vi "战舰+敌机爆炸.vi"() -> ()   [LabVIEW 2018]
panel:
  out "敌机爆炸":picture
  in  "敌机数量":dbl
  in  "敌机速度":dbl
  out "敌机":picture
  out "按键":dbl
  out "战舰":T1
  out "激光武器1":T2
  out "激光武器 2":T2
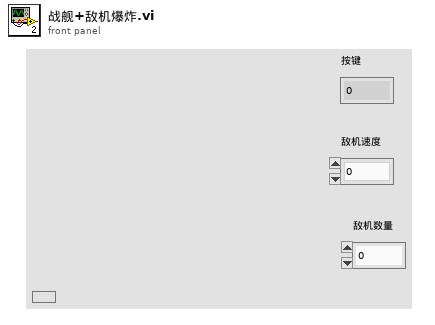
[diagram p1: front panel]
types:
  T1 = typedef "战列巡洋舰.ctl" = picture
  T2 = typedef "战列巡洋舰_激光武器.ctl" = picture
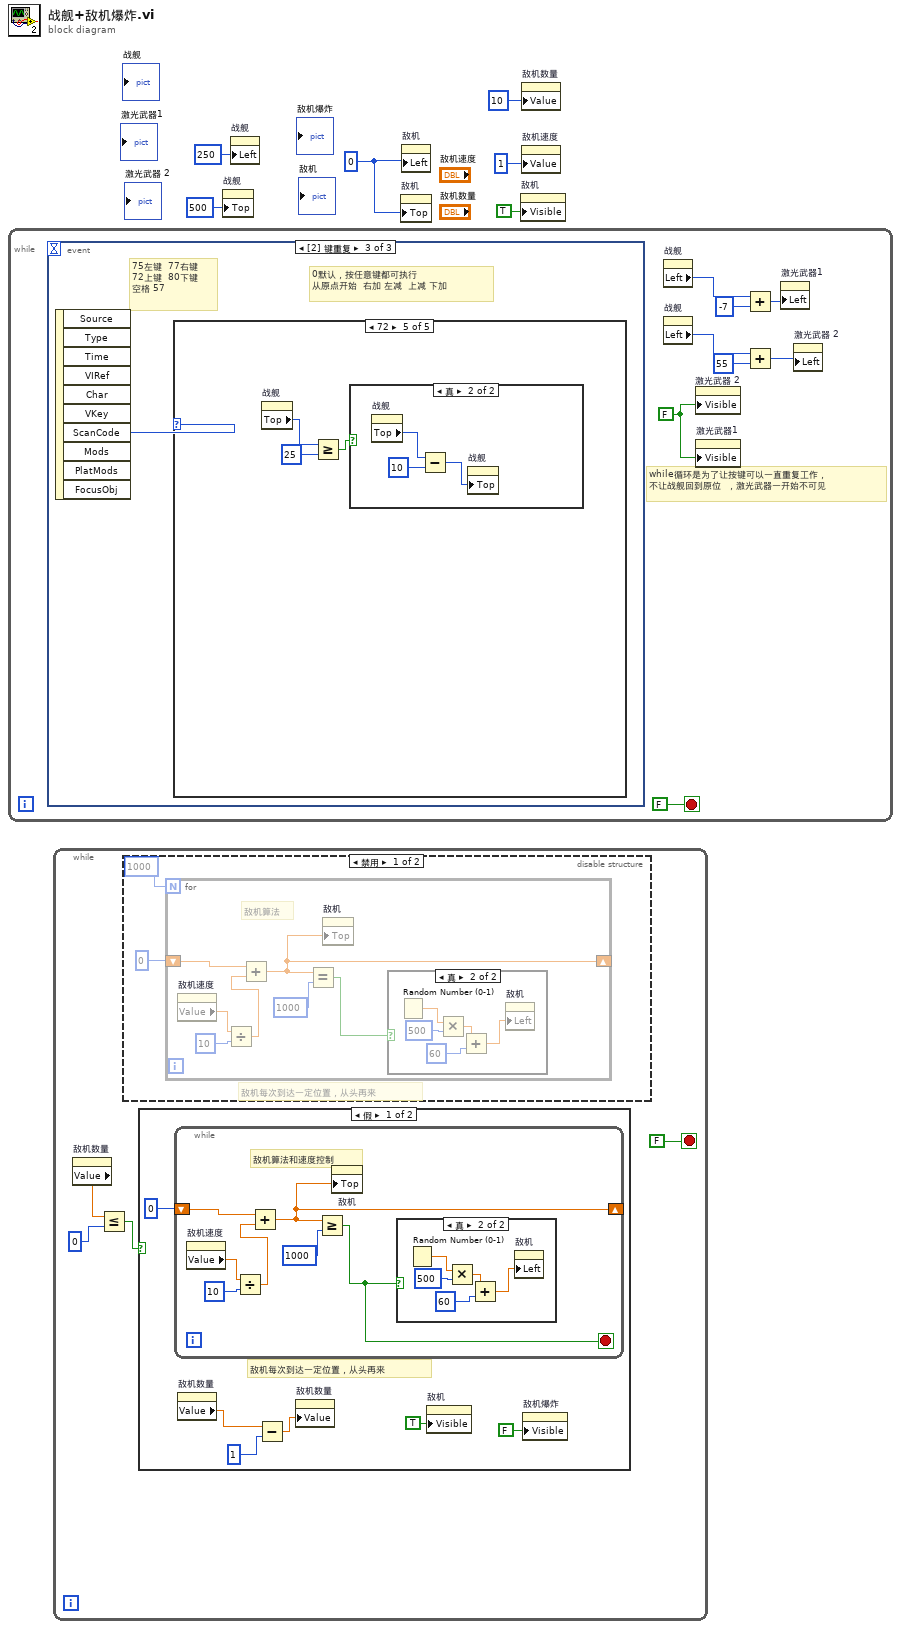
[diagram p0: block diagram]
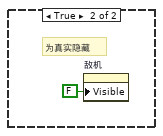
[diagram p3: hidden frame]
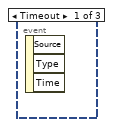
[diagram p6: hidden frame]
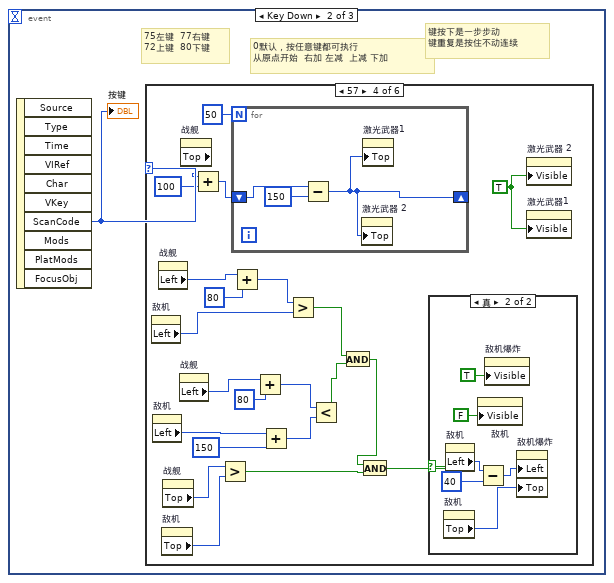
[diagram p7: hidden frame]
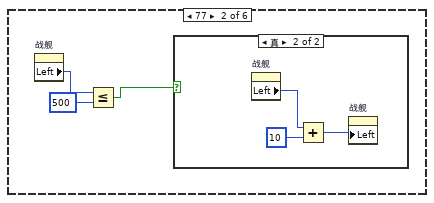
[diagram p9: hidden frame]
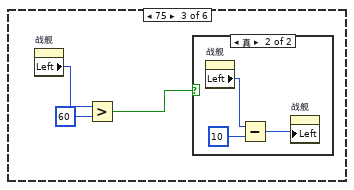
[diagram p11: hidden frame]
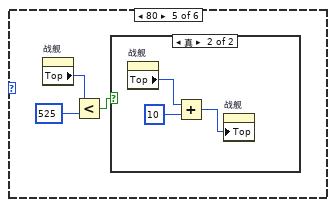
[diagram p14: hidden frame]
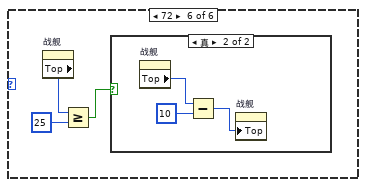
[diagram p16: hidden frame]
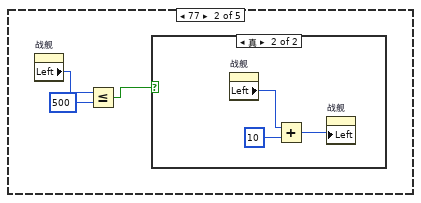
[diagram p19: hidden frame]
diagram:
  w1 = 0
  n1 = while {
    stop <- FALSE stop-if-true
    w7 = FALSE
    # "while循环是为了让按键可以一直重复工作，\n不让战舰回到原位  ，激光武器一开始不可见"
    n2 = event shown="[2] 键重复" {
      selector: _ -> [_ _ _]
      dyn-events: _ -> [_ _ _]
      timeout: _ -> [_ _ _]
      event Timeout {
        n3 = event-data() -> ()  [unwired: 1 in, 3 out]
      }
      event Key Down {
        # "键按下是一步步动\n键重复是按住不动连续"
        # "75左键  77右键\n72上键  80下键"
        # "0默认，按任意键都可执行\n从原点开始  右加 左减  上减 下加"
        n4 = event-data() -> ("ScanCode"=w15:i16)  [unwired: 1 in, 9 out]
        "按键" <- w15
        n5 = case shown="57" w15 {
          frame 0, Default {
          }
          frame 77 {
            n6 = property on="战舰" class="Pict (严格)"() -> ("Left"=w18:i32)  [unwired: 2 in, 2 out]
            n7 = Less Or Equal?(x=w18, y=500) -> (x <= y?=w16:bool)
            n8 = case shown="真" w16 {
              frame False {
              }
              frame True {
                n9 = property on="战舰" class="Pict (严格)"() -> ("Left"=w20:i32)  [unwired: 2 in, 2 out]
                n10 = Add(x=w20, y=10) -> (x+y=w21:i32)
                n11 = property on="战舰" class="Pict (严格)"("Left"=w21) -> ()  [unwired: 2 in, 2 out]
              }
            }
          }
          frame 75 {
            n12 = property on="战舰" class="Pict (严格)"() -> ("Left"=w24:i32)  [unwired: 2 in, 2 out]
            n13 = Greater?(x=w24, y=60) -> (0:w22:bool)
            n14 = case shown="真" w22 {
              frame False {
              }
              frame True {
                n15 = property on="战舰" class="Pict (严格)"() -> ("Left"=w26:i32)  [unwired: 2 in, 2 out]
                n16 = Subtract(x=w26, y=10) -> (x-y=w27:i32)
                n17 = property on="战舰" class="Pict (严格)"("Left"=w27) -> ()  [unwired: 2 in, 2 out]
              }
            }
          }
          frame 57 {
            w45 = TRUE
            n18 = property on="敌机" class="Pict"() -> ("Left"=w42:i32)  [unwired: 2 in, 2 out]
            n19 = property on="敌机" class="Pict"() -> ("Left"=w35:i32)  [unwired: 2 in, 2 out]
            n20 = property on="战舰" class="Pict (严格)"() -> ("Left"=w44:i32)  [unwired: 2 in, 2 out]
            n21 = property on="敌机" class="Pict"() -> ("Top"=w28:i32)  [unwired: 2 in, 2 out]
            n22 = property on="战舰" class="Pict (严格)"() -> ("Top"=w29:i32)  [unwired: 2 in, 2 out]
            n23 = property on="战舰" class="Pict (严格)"() -> ("Left"=w37:i32)  [unwired: 2 in, 2 out]
            n24 = property on="战舰" class="Pict (严格)"() -> ("Top"=w48:i32)  [unwired: 2 in, 2 out]
            n25 = Add(x=w48, y=100) -> (x+y=w46:i32)
            n26 = Greater?(x=w29, y=w28) -> (0:w31:bool)
            n27 = for {
              N: 50 -> [_]
              shift-right: [w56] -> _
              shift-left: w46 -> [w58]
              n28 = Subtract(x=w58, y=150) -> (x-y=w56:i32)
              n29 = property on="激光武器 2" class="Pict (严格)"("Top"=w56) -> ()  [unwired: 2 in, 2 out]
              n30 = property on="激光武器1" class="Pict (严格)"("Top"=w56) -> ()  [unwired: 2 in, 2 out]
            }
            n31 = Add(x=w44, y=80) -> (x+y=w41:i32)
            n32 = Add(x=w37, y=80) -> (x+y=w39:i32)
            n33 = Add(x=w35, y=150) -> (x+y=w34:i32)
            n34 = Greater?(x=w41, y=w42) -> (0:w40:bool)
            n35 = Less?(x=w39, y=w34) -> (x < y?=w36:bool)
            n36 = And(x=w40, y=w36) -> (x .and. y?=w32:bool)
            n37 = And(x=w32, y=w31) -> (x .and. y?=w30:bool)
            n38 = case shown="真" w30 {
              frame False {
              }
              frame True {
                n39 = property on="敌机" class="Pict"() -> ("Top"=w53:i32)  [unwired: 2 in, 2 out]
                n40 = property on="敌机" class="Pict"() -> ("Left"=w51:i32)  [unwired: 2 in, 2 out]
                n41 = property on="敌机" class="Pict"("Visible"=FALSE ("可见")) -> ()  [unwired: 2 in, 2 out]
                n42 = Subtract(x=w51, y=40) -> (x-y=w50:i32)
                n43 = property on="敌机爆炸" class="Pict"("Visible"=TRUE ("可见")) -> ()  [unwired: 2 in, 2 out]
                n44 = property on="敌机爆炸" class="Pict"("Left"=w50, "Top"=w53) -> ()  [unwired: 2 in, 2 out]
              }
            }
            n45 = property on="激光武器 2" class="Pict (严格)"("Visible"=w45) -> ()  [unwired: 2 in, 2 out]
            n46 = property on="激光武器1" class="Pict (严格)"("Visible"=w45) -> ()  [unwired: 2 in, 2 out]
          }
          frame 80 {
            n47 = property on="战舰" class="Pict (严格)"() -> ("Top"=w61:i32)  [unwired: 2 in, 2 out]
            n48 = Less?(x=w61, y=525) -> (x < y?=w59:bool)
            n49 = case shown="真" w59 {
              frame False {
              }
              frame True {
                n50 = property on="战舰" class="Pict (严格)"() -> ("Top"=w63:i32)  [unwired: 2 in, 2 out]
                n51 = Add(x=w63, y=10) -> (x+y=w62:i32)
                n52 = property on="战舰" class="Pict (严格)"("Top"=w62) -> ()  [unwired: 2 in, 2 out]
              }
            }
          }
          frame 72 {
            n53 = property on="战舰" class="Pict (严格)"() -> ("Top"=w67:i32)  [unwired: 2 in, 2 out]
            n54 = Greater Or Equal?(x=w67, y=25) -> (x >= y?=w66:bool)
            n55 = case shown="真" w66 {
              frame False {
              }
              frame True {
                n56 = property on="战舰" class="Pict (严格)"() -> ("Top"=w70:i32)  [unwired: 2 in, 2 out]
                n57 = Subtract(x=w70, y=10) -> (x-y=w69:i32)
                n58 = property on="战舰" class="Pict (严格)"("Top"=w69) -> ()  [unwired: 2 in, 2 out]
              }
            }
          }
        }
      }
      event Key Repeat {
        # "75左键  77右键\n72上键  80下键\n空格 57"
        # "0默认，按任意键都可执行\n从原点开始  右加 左减  上减 下加"
        n59 = event-data() -> ("ScanCode"=w71:i16)  [unwired: 1 in, 9 out]
        n60 = case shown="72" w71 {
          frame 0, Default {
          }
          frame 77 {
            n61 = property on="战舰" class="Pict (严格)"() -> ("Left"=w74:i32)  [unwired: 2 in, 2 out]
            n62 = Less Or Equal?(x=w74, y=500) -> (x <= y?=w73:bool)
            n63 = case shown="真" w73 {
              frame False {
              }
              frame True {
                n64 = property on="战舰" class="Pict (严格)"() -> ("Left"=w76:i32)  [unwired: 2 in, 2 out]
                n65 = Add(x=w76, y=10) -> (x+y=w77:i32)
                n66 = property on="战舰" class="Pict (严格)"("Left"=w77) -> ()  [unwired: 2 in, 2 out]
              }
            }
          }
          frame 75 {
            n67 = property on="战舰" class="Pict (严格)"() -> ("Left"=w80:i32)  [unwired: 2 in, 2 out]
            n68 = Greater Or Equal?(x=w80, y=25) -> (x >= y?=w79:bool)
            n69 = case shown="真" w79 {
              frame False {
              }
              frame True {
                n70 = property on="战舰" class="Pict (严格)"() -> ("Left"=w83:i32)  [unwired: 2 in, 2 out]
                n71 = Subtract(x=w83, y=10) -> (x-y=w82:i32)
                n72 = property on="战舰" class="Pict (严格)"("Left"=w82) -> ()  [unwired: 2 in, 2 out]
              }
            }
          }
          frame 80 {
            n73 = property on="战舰" class="Pict (严格)"() -> ("Top"=w86:i32)  [unwired: 2 in, 2 out]
            n74 = Less Or Equal?(x=w86, y=525) -> (x <= y?=w85:bool)
            n75 = case shown="真" w85 {
              frame False {
              }
              frame True {
                n76 = property on="战舰" class="Pict (严格)"() -> ("Top"=w88:i32)  [unwired: 2 in, 2 out]
                n77 = Add(x=w88, y=10) -> (x+y=w87:i32)
                n78 = property on="战舰" class="Pict (严格)"("Top"=w87) -> ()  [unwired: 2 in, 2 out]
              }
            }
          }
          frame 72 {
            n79 = property on="战舰" class="Pict (严格)"() -> ("Top"=w92:i32)  [unwired: 2 in, 2 out]
            n80 = Greater Or Equal?(x=w92, y=25) -> (x >= y?=w91:bool)
            n81 = case shown="真" w91 {
              frame False {
              }
              frame True {
                n82 = property on="战舰" class="Pict (严格)"() -> ("Top"=w95:i32)  [unwired: 2 in, 2 out]
                n83 = Subtract(x=w95, y=10) -> (x-y=w94:i32)
                n84 = property on="战舰" class="Pict (严格)"("Top"=w94) -> ()  [unwired: 2 in, 2 out]
              }
            }
          }
        }
      }
    }
    n85 = property on="战舰" class="Pict (严格)"() -> ("Left"=w13:i32)  [unwired: 2 in, 2 out]
    n86 = property on="战舰" class="Pict (严格)"() -> ("Left"=w9:i32)  [unwired: 2 in, 2 out]
    n87 = property on="激光武器 2" class="Pict (严格)"("Visible"=w7) -> ()  [unwired: 2 in, 2 out]
    n88 = property on="激光武器1" class="Pict (严格)"("Visible"=w7) -> ()  [unwired: 2 in, 2 out]
    n89 = Add(x=w13, y=-7) -> (x+y=w12:i32)
    n90 = Add(x=w9, y=55) -> (x+y=w8:i32)
    n91 = property on="激光武器1" class="Pict (严格)"("Left"=w12) -> ()  [unwired: 2 in, 2 out]
    n92 = property on="激光武器 2" class="Pict (严格)"("Left"=w8) -> ()  [unwired: 2 in, 2 out]
  }
  n93 = while {
    stop <- FALSE stop-if-true
    n94 = property on="敌机数量" class="DigNum (严格)"() -> ("Value"=w98:dbl)  [unwired: 2 in, 2 out]
    n95 = Less Or Equal?(x=w98, y=0) -> (x <= y?=w97:bool)
    n96 = disable-structure shown="禁用" {
      frame Disabled {
        # "敌机每次到达一定位置，从头再来"
        n97 = for {
          N: 1000 -> [_]
          shift-right: [w124] -> _
          shift-left: 0 -> [w127]
          # "敌机算法"
          n98 = property on="敌机速度" class="DigNum (严格)"() -> ("Value"=w123:dbl)  [unwired: 2 in, 2 out]
          n99 = Divide(x=w123, y=10) -> (x/y=w122:dbl)
          n100 = Add(x=w127, y=w122) -> (x+y=w124:dbl)
          n101 = Equal?(x=w124, y=1000) -> (x = y?=w125:bool)
          n102 = property on="敌机" class="Pict"("Top"=w124) -> ()  [unwired: 2 in, 2 out]
          n103 = case shown="真" w125 {
            frame False {
            }
            frame True {
              n104 = Random Number (0-1)() -> (number: 0 to 1=w132:dbl)
              n105 = Multiply(x=w132, y=500) -> (x*y=w130:dbl)
              n106 = Add(x=w130, y=60) -> (x+y=w129:dbl)
              n107 = property on="敌机" class="Pict"("Left"=w129) -> ()  [unwired: 2 in, 2 out]
            }
          }
        }
      }
      frame Enabled {
      }
    }
    n108 = case shown="假" w97 {
      frame False {
        # "敌机每次到达一定位置，从头再来"
        n109 = while {
          shift-right: [w110] -> _
          shift-left: 0 -> [w112]
          stop <- w106 stop-if-true
          # "敌机算法和速度控制"
          n110 = property on="敌机速度" class="DigNum (严格)"() -> ("Value"=w109:dbl)  [unwired: 2 in, 2 out]
          n111 = Divide(x=w109, y=10) -> (x/y=w108:dbl)
          n112 = Add(x=w112, y=w108) -> (x+y=w110:dbl)
          n113 = Greater Or Equal?(x=w110, y=1000) -> (x >= y?=w106:bool)
          n114 = property on="敌机" class="Pict"("Top"=w110) -> ()  [unwired: 2 in, 2 out]
          n115 = case shown="真" w106 {
            frame False {
            }
            frame True {
              n116 = Random Number (0-1)() -> (number: 0 to 1=w117:dbl)
              n117 = Multiply(x=w117, y=500) -> (x*y=w115:dbl)
              n118 = Add(x=w115, y=60) -> (x+y=w114:dbl)
              n119 = property on="敌机" class="Pict"("Left"=w114) -> ()  [unwired: 2 in, 2 out]
            }
          }
        }
        n120 = property on="敌机数量" class="DigNum (严格)"() -> ("Value"=w103:dbl)  [unwired: 2 in, 2 out]
        n121 = Subtract(x=w103, y=1) -> (x-y=w104:dbl)
        n122 = property on="敌机数量" class="DigNum (严格)"("Value"=w104) -> ()  [unwired: 2 in, 2 out]
        n123 = property on="敌机" class="Pict"("Visible"=TRUE ("可见")) -> ()  [unwired: 2 in, 2 out]
        n124 = property on="敌机爆炸" class="Pict"("Visible"=FALSE ("可见")) -> ()  [unwired: 2 in, 2 out]
      }
      frame True {
        # "为真实隐藏"
        n125 = property on="敌机" class="Pict"("Visible"=FALSE ("可见")) -> ()  [unwired: 2 in, 2 out]
      }
    }
  }
  n126 = property on="战舰" class="Pict (严格)"("Top"=500 ("位置:置顶")) -> ()  [unwired: 2 in, 2 out]
  n127 = property on="战舰" class="Pict (严格)"("Left"=250 ("位置:居左")) -> ()  [unwired: 2 in, 2 out]
  n128 = property on="敌机" class="Pict"("Top"=w1) -> ()  [unwired: 2 in, 2 out]
  n129 = property on="敌机" class="Pict"("Left"=w1) -> ()  [unwired: 2 in, 2 out]
  n130 = property on="敌机" class="Pict"("Visible"=TRUE ("可见")) -> ()  [unwired: 2 in, 2 out]
  n131 = property on="敌机数量" class="DigNum (严格)"("Value"=10) -> ()  [unwired: 2 in, 2 out]
  n132 = property on="敌机速度" class="DigNum (严格)"("Value"=1) -> ()  [unwired: 2 in, 2 out]
